vi "runscenario string to items.vi"(1 "value":string) -> (0 "Items":T1[](array[typedef]))   [LabVIEW 2011]
uses:
  _cgi-lib/TDM_INDEX Record.ctl
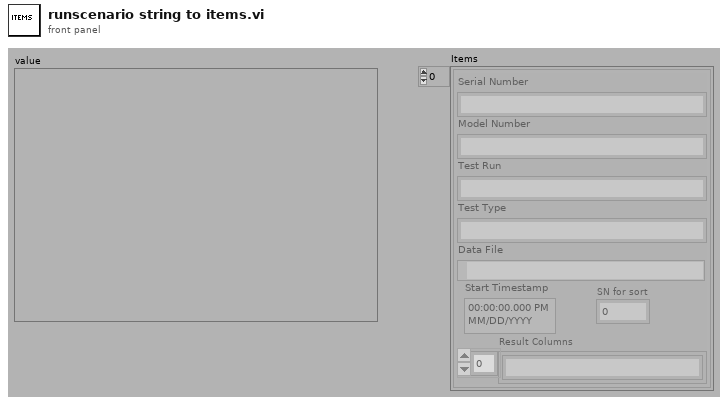
[diagram p1: front panel]
types:
  T1 = typedef "TDM_INDEX Record.ctl" = cluster{"Model Number":string, "SN for sort":i32, "Test Type":string, "Test Run":string, "Serial Number":string, "Start Timestamp":timestamp, "Data File":path, "Result Columns":string[]}
  T2 = cluster{"[0]":string, "[1]":string, "[2]":string, "[3]":string, "[4]":string}
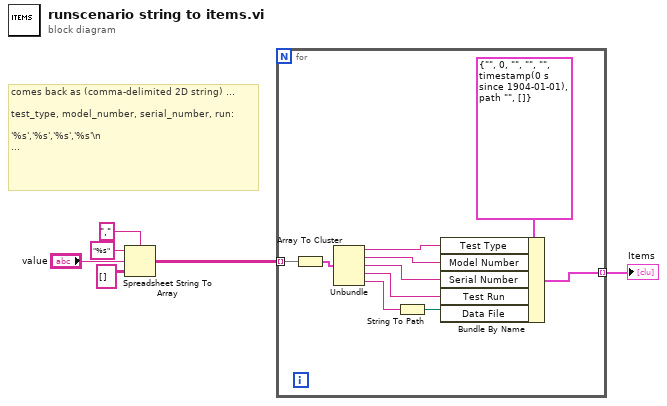
[diagram p0: block diagram]
diagram:
  # "comes back as (comma-delimited 2D string) ...\n\ntest_type, model_number, serial_number, run:\n\n'%s','%s','%s','%s'\\n\n..."
  n1 = Spreadsheet String To Array(delimiter (Tab)=",", format string="%s" ("Template (\"\")"), spreadsheet string="value", array type (2D Dbl)=string[][] []) -> (array=w5:string[][])
  n2 = for {
    tunnel: w5 -> [w14] mode=indexing
    tunnel: [w15] -> w6 mode=indexing
    n3 = Array To Cluster(array=w14) -> (cluster=w13:T2)
    n4 = Unbundle(w13) -> ("[0]"=w9:string, "[1]"=w10:string, "[2]"=w11:string, "[3]"=w12:string, "[4]"=w8:string)
    n5 = String To Path(string=w8) -> (path=w7:path)
    n6 = Bundle By Name(cluster=T1 {"Model Number"="", "SN for sort"=0, "Test Type"="", "Test Run"="", "Serial Number"="", "Start Timestamp"=timestamp(0 s since 1904-01-01), "Data File"=path "", "Result Columns"=[]} ("TDM_INDEX Record"), "Test Type"=w9, "Model Number"=w10, "Serial Number"=w11, "Test Run"=w12, "Data File"=w7) -> (w15:T1)
  }
  "Items" <- w6
